vi "AddError.vi"(6 "NoErrorMessage":string="Vac OK", 7 "ErrorMessage":string="Unexpectced vacuum state. There might be a leak.", 8 "error in":errorcluster, 10 "code":i32=-999, 11 "Error?":bool) -> (0 "Error out":errorcluster)   [LabVIEW 2019]
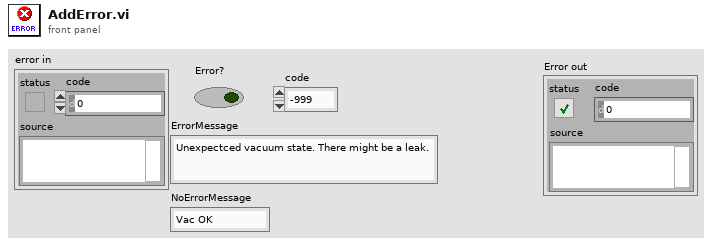
[diagram p1: front panel]
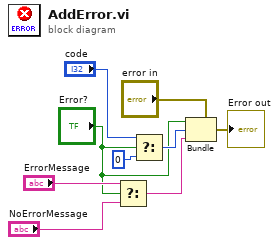
[diagram p0: block diagram]
diagram:
  n1 = Select(t="ErrorMessage", s="Error?", f="NoErrorMessage") -> (s? t:f=w7:string)
  n2 = Select(t="code", s="Error?", f=0) -> (s? t:f=w2:i32)
  n3 = Bundle(cluster="error in", "status"="Error?", "code"=w2, "source"=w7) -> (→"Error out":errorcluster)
